vi "rt.vi"() -> ()   [LabVIEW 2019]
uses:
  controls/sm_cluster.ctl
  lib/labviewRT-EPICS/sm double read and increment.vi
  lib/labviewRT-EPICS/sm string write and increment.vi
  lib/labviewRT-EPICS/sm i64 read and increment.vi
  lib/labviewRT-EPICS/sm string read and increment.vi
  lib/labviewRT-EPICS/sm u32 write and increment.vi
  lib/labviewRT-EPICS/sm u64 read and increment.vi
  lib/labviewRT-EPICS/linuxSharedMemory.lvlib
panel:
  out "u64_7":u64
  in  "stringin6":string
  in  "u32_5":u32
  out "stringout4":string
  out "i64_3":i64
  out "double 1":dbl format="%#.40f"
  in  "stringin2":string
  out "Shared memory cluster output":T1
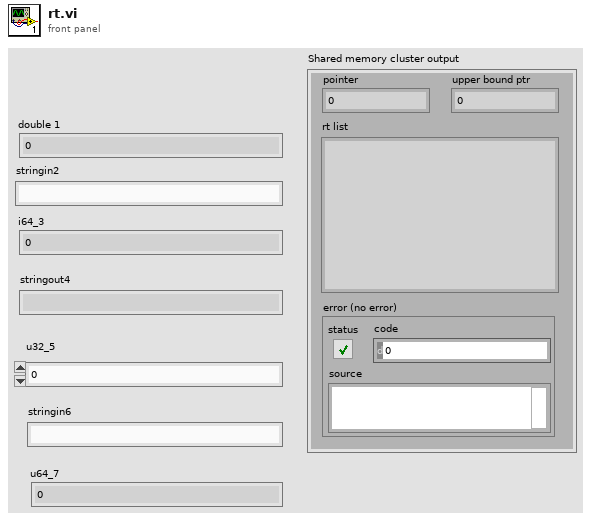
[diagram p1: front panel]
types:
  T1 = typedef "linuxSharedMemory.lvlib/sm_cluster.ctl" = cluster{"rt list":string, "error (no error)":errorcluster, "pointer":u64, "upper bound ptr":u64}
  T2 = typedef "Linux RT IPC.Shared Memory.lvlib/reference.ctl" = refnum<data-value>
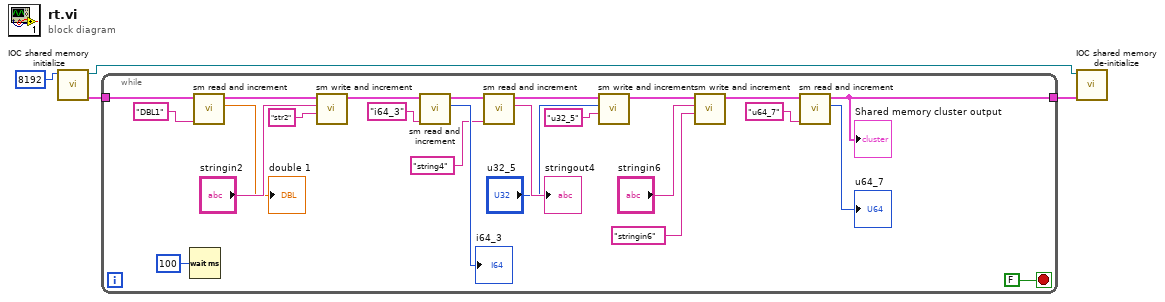
[diagram p0: block diagram]
diagram:
  n1 = call "IOC shared memory initialize.vi"("Shared Memory Size (bytes)"=8192) -> ("Shared memory cluster"=w3:T1, "shared memory class"=w4:T2)  [unwired: 9 in]
  n2 = while {
    tunnel: w3 -> [w28]
    tunnel: [w21] -> w2
    stop <- FALSE stop-if-true
    n3 = Wait (ms)(milliseconds to wait=u32 100) -> ()  [unwired: 1 out]
    n4 = call-poly "sm read and increment.vi"("Identifier"="DBL1", "Shared memory cluster input"=w28) -> ("Value out"=→"double 1":dbl, "Shared memory cluster output"=w27:T1)  [unwired: 8 in]
    n5 = call-poly "sm write and increment.vi"("Identifier"="str2", "String in"="stringin2", "Shared memory cluster input"=w27) -> ("Shared memory cluster output"=w26:T1)  [unwired: 8 in]
    n6 = call-poly "sm read and increment.vi"("Identifier"="i64_3", "Shared memory cluster input"=w26) -> ("Value out"=→"i64_3":i64, "Shared memory cluster output"=w25:T1)  [unwired: 8 in]
    n7 = call-poly "sm read and increment.vi"("Identifier"="string4", "Shared memory cluster"=w25) -> ("String out"=→"stringout4":string, "Shared memory cluster output"=w24:T1)  [unwired: 8 in]
    n8 = call-poly "sm write and increment.vi"("Identifier"="u32_5", "value in"="u32_5", "Shared memory cluster input"=w24) -> ("Shared memory cluster output"=w23:T1)  [unwired: 8 in]
    n9 = call-poly "sm write and increment.vi"("Identifier"="stringin6", "String in"="stringin6", "Shared memory cluster input"=w23) -> ("Shared memory cluster output"=w22:T1)  [unwired: 8 in]
    n10 = call-poly "sm read and increment.vi"("Identifier"="u64_7", "Shared memory cluster input"=w22) -> ("Value out"=→"u64_7":u64, "Shared memory cluster output"=w21:T1)  [unwired: 8 in]
    "Shared memory cluster output" <- w21
  }
  n11 = call "IOC shared memory de-initialize.vi"("shared memory in"=w4, "Shared memory cluster"=w2) -> ()  [unwired: 9 in]
